vi "Write instrSplitters.vi"(8 "error in (no error)":errorcluster, 10 "Splitters":refnum<vi>[](array[refnum]), 11 "Manual UI in":refnum<class "Manual UI.lvclass">) -> (0 "error out":errorcluster, 3 "Manual UI out":refnum<class "Manual UI.lvclass">)   [LabVIEW 2023, in "Manual UI.lvlib" / "Manual UI.lvclass"]
uses:
  Project/Manual UI.lvclass
  Project/Manual UI.lvclass/Manual UI.ctl
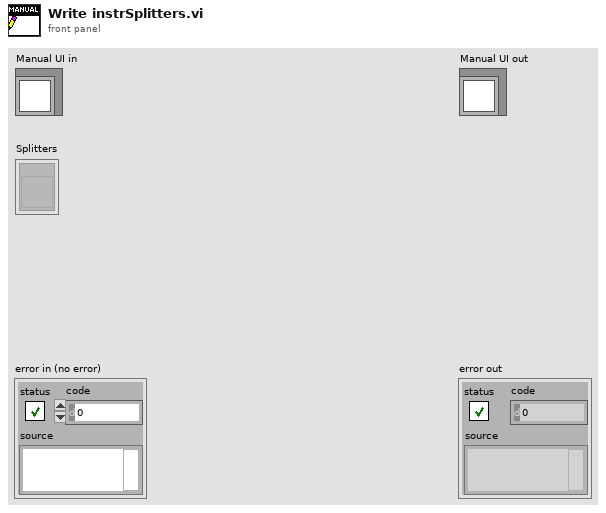
[diagram p1: front panel]
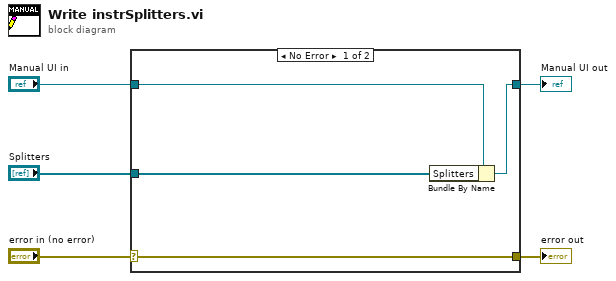
[diagram p0: block diagram]
diagram:
  n1 = case shown="No Error" "error in (no error)" {
    selector: "error in (no error)" -> [w9 w10]
    tunnel: [w9 w10] -> w4
    tunnel: [w7 w11] -> w2
    tunnel: "Manual UI in" -> [w8 w11]
    tunnel: "Splitters" -> [w6 _]
    frame No Error {
      n2 = Bundle By Name(cluster=w8, "Splitters"=w6) -> (w7:refnum<class "Manual UI.lvclass">)
    }
    frame Error {
    }
  }
  "error out" <- w4
  "Manual UI out" <- w2
